vi "S30c_dll F66.vi"(4 "error in":errorcluster, 6 "New address":u8, 7 "Dev Addr":u8=250) -> (0 "error out":errorcluster, 2 "Actual address":u8)   [LabVIEW 2014, in "K_S30c_dll.lvlib"]
uses:
  K_S30c_dll.lvlib
  s30c.dll
panel:
  # "Function 66: Read / set device address \n\nusing s30c.dll\nKeller AG für Druckmesstechnik, 29.5.08 b.v."
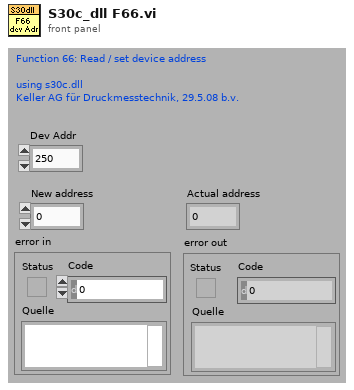
[diagram p1: front panel]
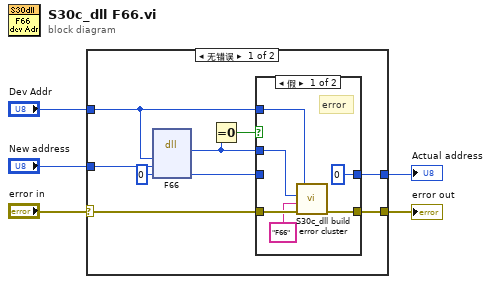
[diagram p0: block diagram]
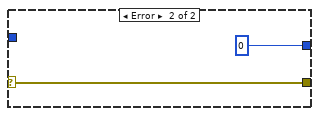
[diagram p3: hidden frame]
diagram:
  n1 = case shown="无错误" "error in" {
    selector: "error in" -> [w10 w24]
    tunnel: [w13 w24] -> w3
    tunnel: "Dev Addr" -> [w11 _]
    tunnel: "New address" -> [w9 _]
    tunnel: [w6 u8 0 ("ActAdress")] -> w2
    frame No Error {
      n2 = dll-call lib="PTH2Labs EworkSINOPEC北控自动相渗software2.08.5_dlls30c.dll" fn="F66"("DevAddr"=w11, "New Addr"=w9, "ActAdress"=u8 0) -> (w8:i16, "ActAdress"=w7:u8)  [unwired: 5 in, 2 out]
      n3 = Equal To 0?(x=w8) -> (x = 0?=w14:bool)
      n4 = case shown="假" w14 {
        tunnel: w10 -> [w20 w22]
        tunnel: [w19 w22] -> w13
        tunnel: w11 -> [w17 _]
        tunnel: w8 -> [w16 _]
        tunnel: w7 -> [_ w21]
        tunnel: [u8 0 ("ActAdress") w21] -> w6
        frame False {
          # "error"
          n5 = call "S30c_dll build error cluster.vi"("error in"=w20, "error Text"="F66", "error code"=w16, "Dev Addr"=w17) -> ("error out"=w19:errorcluster)  [unwired: 3 in]
        }
        frame True {
        }
      }
    }
    frame Error {
    }
  }
  "error out" <- w3
  "Actual address" <- w2
